vi "replaceElementValue.vi"(7 "replaceElementIn":string, 8 "error in (no error)":errorcluster, 9 "replaceWithValue":string, 10 "replacementElementName":string, 11 "xmlNode in":refnum<class "xmlNode.lvclass">) -> (0 "error out":errorcluster, 1 "found?":bool=TRUE, 2 "replacementxXmlNode":refnum<class "xmlNode.lvclass">, 3 "xmlNode out":refnum<class "xmlNode.lvclass">)   [LabVIEW 2009, in "Tools.lvlib" / "xml.lvlib" / "xmlNode.lvclass"]
uses:
  xmlNode.lvclass
  XmlParser.lvclass
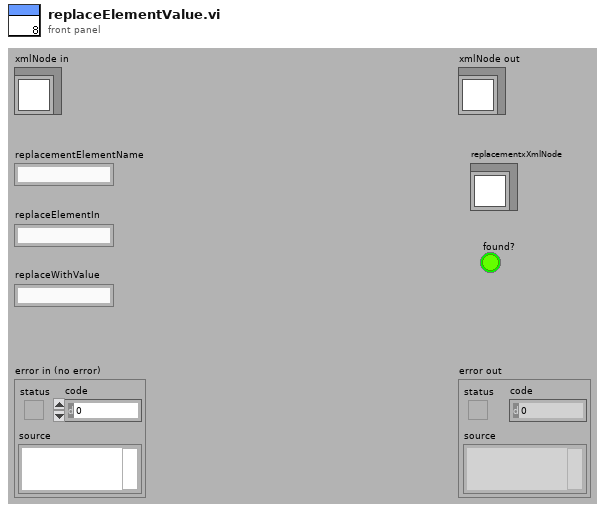
[diagram p1: front panel]
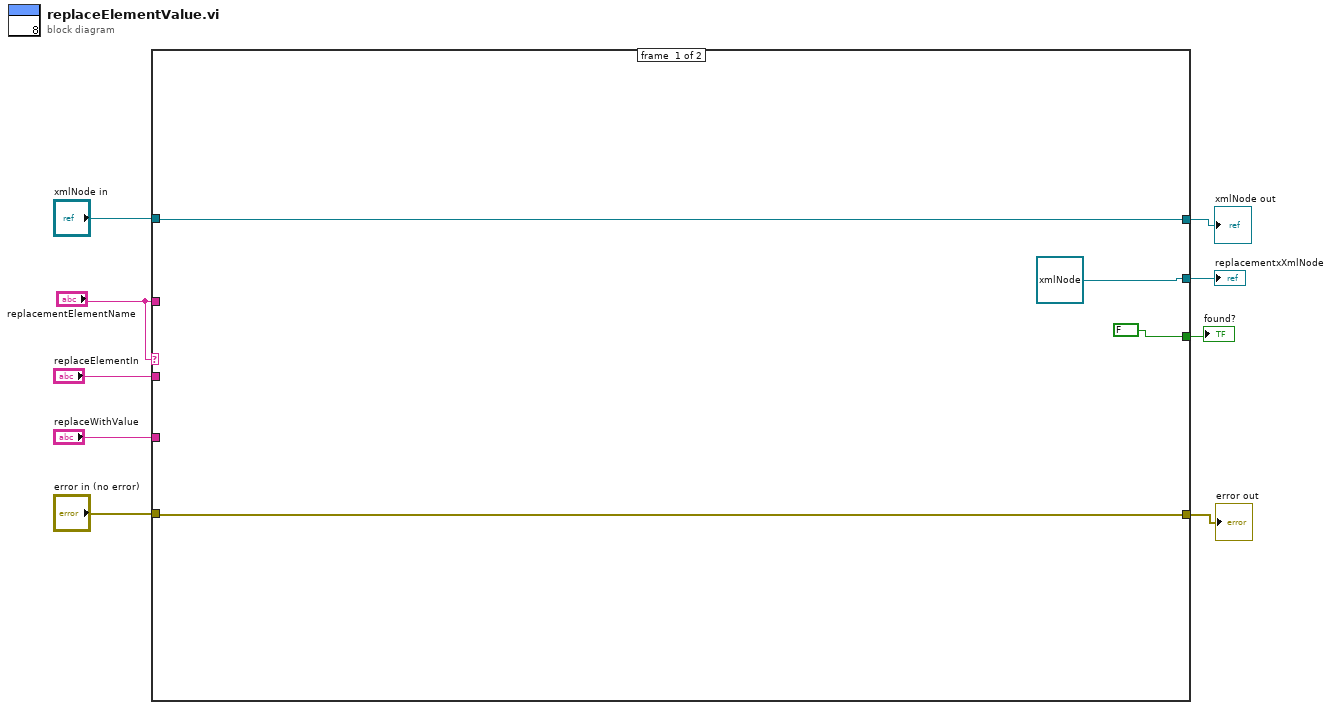
[diagram p0: block diagram]
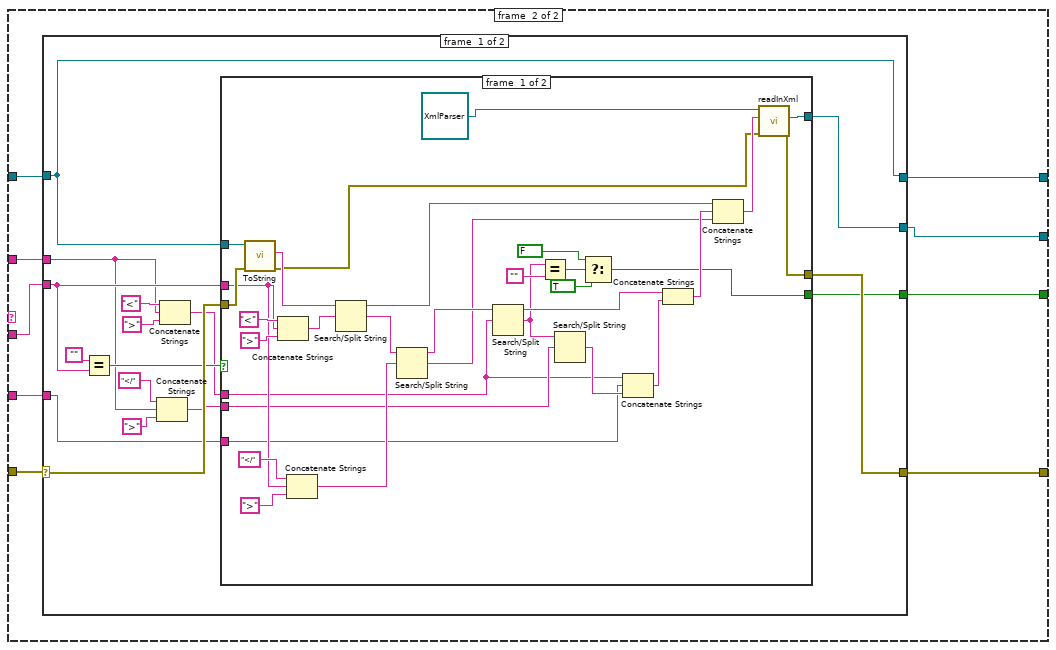
[diagram p2: hidden frame]
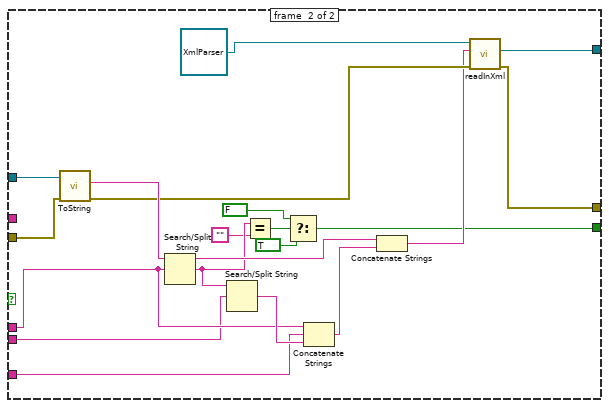
[diagram p3: hidden frame]
diagram:
  n1 = case shown="Default" "replacementElementName" {
    tunnel: "error in (no error)" -> [w10 w22]
    tunnel: "xmlNode in" -> [w13 w21]
    tunnel: "replaceElementIn" -> [_ w20]
    tunnel: "replacementElementName" -> [_ w19]
    tunnel: "replaceWithValue" -> [_ w18]
    tunnel: [w13 w17] -> w4
    tunnel: [refnum<class "xmlNode.lvclass"> refnum ("Tools.lvlib:xml.lvlib:xmlNode.lvclass") w16] -> w3
    tunnel: [FALSE w15] -> w2
    tunnel: [w10 w14] -> w1
    frame #0 {
    }
    frame #1 {
      n2 = case shown="No Error" w22 {
        selector: w22 -> [w37 w92]
        tunnel: [w24 w92] -> w14
        tunnel: [w38 w91] -> w17
        tunnel: w21 -> [w38 w91]
        tunnel: w20 -> [w36 _]
        tunnel: w19 -> [w31 _]
        tunnel: w18 -> [w26 _]
        tunnel: [w25 _] -> w16
        tunnel: [w23 _] -> w15
        frame #0 {
          n3 = Equal?(x="", y=w36) -> (x = y?=w32:bool)
          n4 = Concatenate Strings("</", w31, ">") -> (w27:string)
          n5 = Concatenate Strings("<", w31, ">") -> (w28:string)
          n6 = case shown="False" w32 {
            tunnel: w38 -> [w70 w90]
            tunnel: w37 -> [w69 w89]
            tunnel: w36 -> [w57 _]
            tunnel: [w46 w79] -> w24
            tunnel: w28 -> [w53 w85]
            tunnel: w27 -> [w54 w84]
            tunnel: w26 -> [w52 w83]
            tunnel: [w45 w78] -> w25
            tunnel: [w40 w71] -> w23
            frame #0 {
              n7 = call-dynamic "ToString.vi"("error in (no error)"=w69, "xmlNode in"=w70) -> ("error out"=w47:errorcluster, "xml"=w68:string)  [unwired: 7 in, 1 out]
              n8 = Concatenate Strings("<", w57, ">") -> (w65:string)
              n9 = Concatenate Strings("</", w57, ">") -> (w55:string)
              n10 = Search/Split String(string=w68, search string/char (-)=w65) -> (substring before match=w60:string, match + rest of string=w56:string)  [unwired: 1 in, 1 out]
              n11 = Search/Split String(string=w56, search string/char (-)=w55) -> (substring before match=w51:string, match + rest of string=w49:string)  [unwired: 1 in, 1 out]
              n12 = Search/Split String(string=w51, search string/char (-)=w53) -> (substring before match=w61:string, match + rest of string=w41:string)  [unwired: 1 in, 1 out]
              n13 = Equal?(x=w41, y="") -> (x = y?=w43:bool)
              n14 = Search/Split String(string=w41, search string/char (-)=w54) -> (match + rest of string=w62:string)  [unwired: 1 in, 2 out]
              n15 = Select(t=FALSE, s=w43, f=TRUE) -> (s? t:f=w40:bool)
              n16 = Concatenate Strings(w53, w52, w62) -> (w63:string)
              n17 = Concatenate Strings(w61, w63) -> (w50:string)
              n18 = Concatenate Strings(w60, w50, w49) -> (w48:string)
              n19 = call "readInXml.vi"("error in (no error)"=w47, "xmlString"=w48, "XmlParser in"=refnum<class "XmlParser.lvclass"> refnum ("Tools.lvlib:XmlParser.lvclass")) -> ("error out"=w46:errorcluster, "xmlNode"=w45:refnum<class "xmlNode.lvclass">)  [unwired: 6 in, 1 out]
            }
            frame #1 {
              n20 = call-dynamic "ToString.vi"("error in (no error)"=w89, "xmlNode in"=w90) -> ("error out"=w81:errorcluster, "xml"=w86:string)  [unwired: 7 in, 1 out]
              n21 = Search/Split String(string=w86, search string/char (-)=w85) -> (substring before match=w77:string, match + rest of string=w76:string)  [unwired: 1 in, 1 out]
              n22 = Search/Split String(string=w76, search string/char (-)=w84) -> (match + rest of string=w87:string)  [unwired: 1 in, 2 out]
              n23 = Equal?(x=w76, y="") -> (x = y?=w74:bool)
              n24 = Select(t=FALSE, s=w74, f=TRUE) -> (s? t:f=w71:bool)
              n25 = Concatenate Strings(w85, w83, w87) -> (w88:string)
              n26 = Concatenate Strings(w77, w88) -> (w80:string)
              n27 = call "readInXml.vi"("error in (no error)"=w81, "xmlString"=w80, "XmlParser in"=refnum<class "XmlParser.lvclass"> refnum ("Tools.lvlib:XmlParser.lvclass")) -> ("error out"=w79:errorcluster, "xmlNode"=w78:refnum<class "xmlNode.lvclass">)  [unwired: 6 in, 1 out]
            }
          }
        }
        frame #1 {
        }
      }
    }
  }
  "error out" <- w1
  "xmlNode out" <- w4
  "replacementxXmlNode" <- w3
  "found?" <- w2
